vi "Power of 10.vi"(11 "size":i32) -> (3 "power of 10":i32)   [LabVIEW 2017, in "DSF System Explorer.lvlib"]
uses:
  DSF System Explorer.lvlib
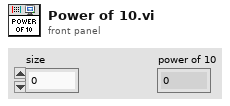
[diagram p1: front panel]
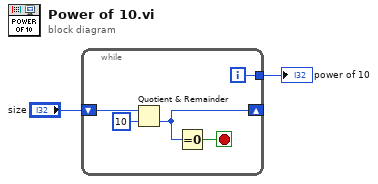
[diagram p0: block diagram]
diagram:
  n1 = while {
    shift-right: [w5] -> _
    shift-left: "size" -> [w7]
    tunnel: [w3] -> w1
    i -> [w3]
    stop <- w4 stop-if-true
    n2 = Quotient & Remainder(x=w7, y=10) -> (floor(x/y)=w5:i32)  [unwired: 1 out]
    n3 = Equal To 0?(x=w5) -> (x = 0?=w4:bool)
  }
  "power of 10" <- w1
